vi "FindAngleDifference.vi"(10 "AngleEncoder":dbl, 11 "AngleSetpoint":dbl) -> (3 "Distance/DirectionOfTurn":dbl)   [LabVIEW 2018]
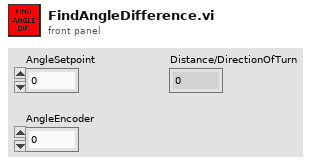
[diagram p1: front panel]
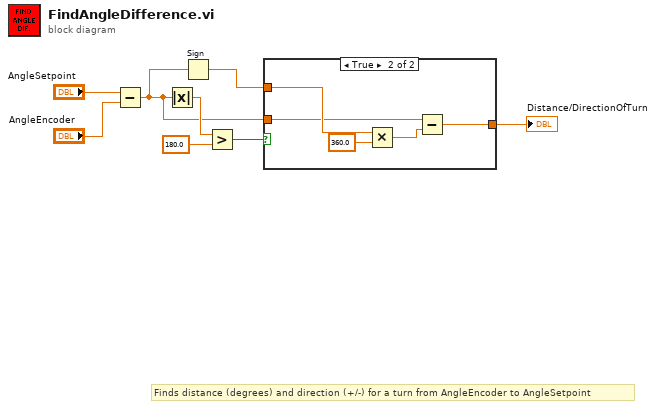
[diagram p0: block diagram]
diagram:
  # "Finds distance (degrees) and direction (+/-) for a turn from AngleEncoder to AngleSetpoint"
  n1 = Subtract(x="AngleSetpoint", y="AngleEncoder") -> (x-y=w1:dbl)
  n2 = Absolute Value(x=w1) -> (abs(x)=w2:dbl)
  n3 = Sign(1:w1) -> (0:w3:dbl)
  n4 = Greater?(x=w2, y=180.0) -> (0:w4:bool)
  n5 = case shown="True" w4 {
    tunnel: w3 -> [_ w14]
    tunnel: [w9 w11] -> w6
    tunnel: w1 -> [w9 w10]
    frame False {
    }
    frame True {
      n6 = Multiply(x=w14, y=360.0) -> (x*y=w12:dbl)
      n7 = Subtract(x=w10, y=w12) -> (x-y=w11:dbl)
    }
  }
  "Distance/DirectionOfTurn" <- w6
